vi "OLED.vi"() -> ()   [LabVIEW 2017]
uses:
  EnumEstados1.ctl
  <vilib>/Analysis/3filter.llb/Filter Passband Type.ctl
  <vilib>/Analysis/baseanly.llb/IIR Cascade Filter (DBL).vi
  <vilib>/Analysis/NI_AALBase.lvlib
panel:
  in  "Reiniciar":bool caption="Blank Button"
  in  "order":i32
  in  "Stop Button":bool
  in  "Save Button":bool
  in  "Guardar en:":path
  out "Voltage-Current Characterization:":cluster{dbl[], "Filtered X":dbl[]}(graph)
  in  "Ok":bool
  out "Voltaje de corte":dbl
  in  "Voltaje final:":dbl=5.0
  in  "Voltaje inicial:":dbl
  in  "Paso":dbl=0.1
  # "OLED"
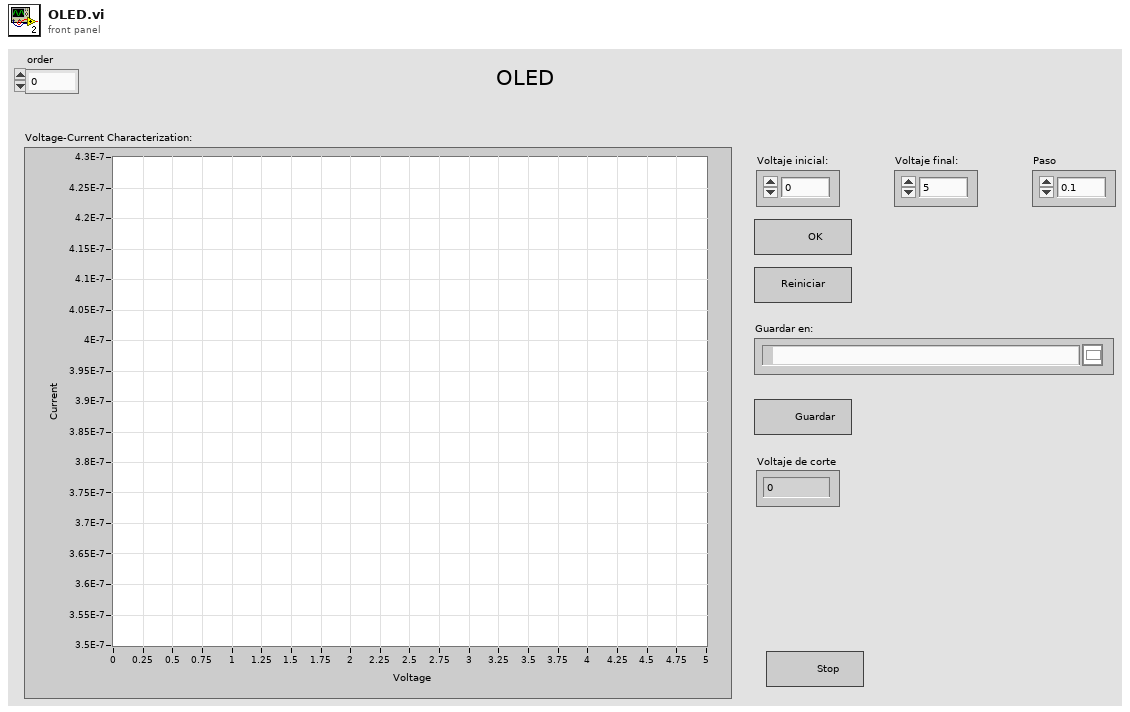
[diagram p1: front panel]
types:
  T1 = typedef "EnumEstados1.ctl" = enum16{"Inicio", "LecturaDatos", "Cierre"}
  T2 = typedef "NI_AALBase.lvlib/Filter Passband Type.ctl" = enum32{"Lowpass", "Highpass", "Bandpass", "Bandstop"}
  T3 = cluster{"task out":refnum<k21>, "error out":errorcluster}
  T4 = cluster{"filter structure":enum32{"IIR 2nd Order", "IIR 4th Order"}, "Reverse Coefficients":dbl[], "Forward Coefficients":dbl[]}
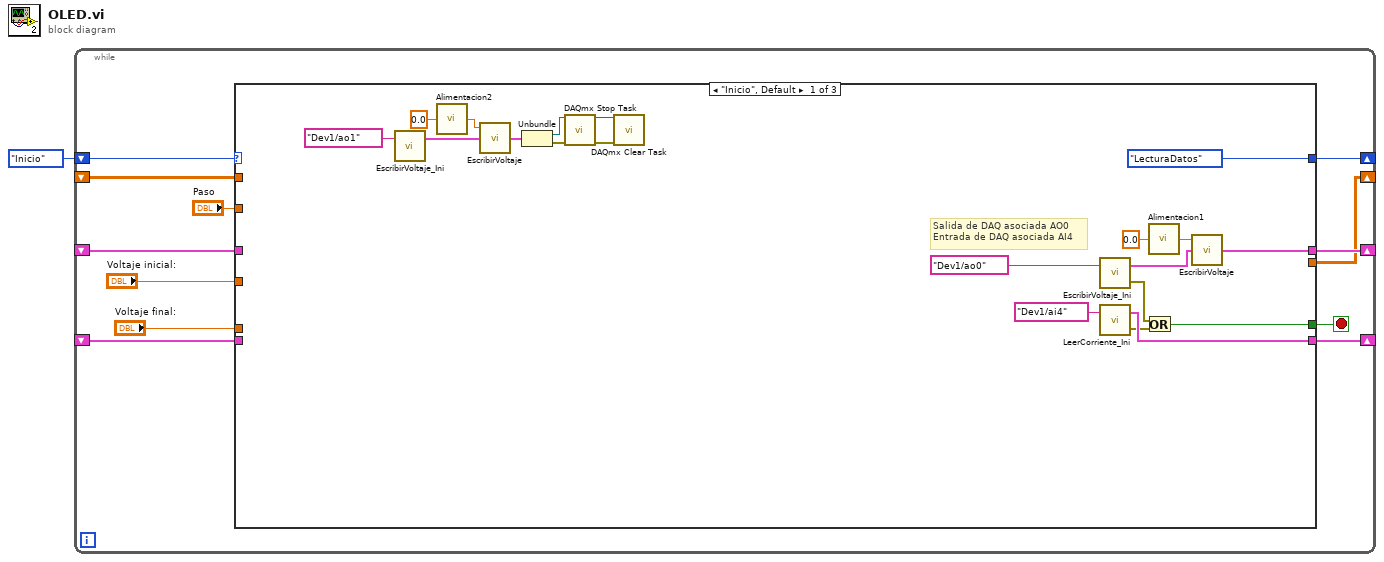
[diagram p0: block diagram]
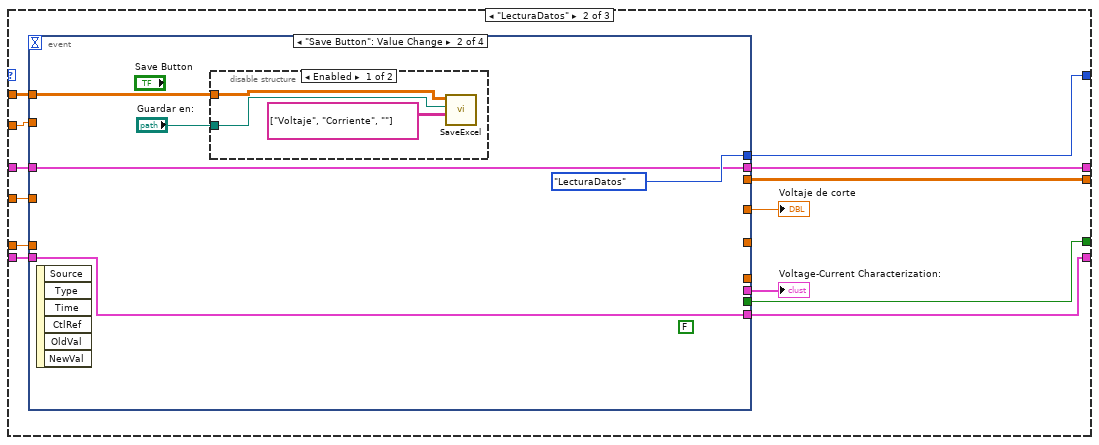
[diagram p2: hidden frame]
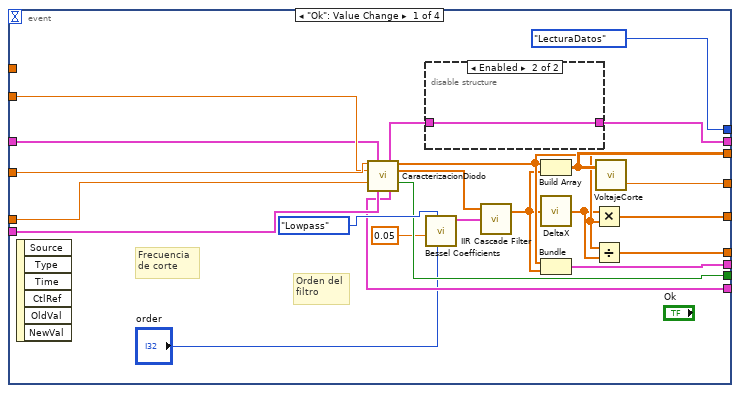
[diagram p3: hidden frame]
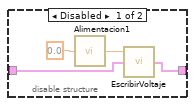
[diagram p4: hidden frame]
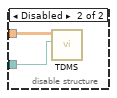
[diagram p5: hidden frame]
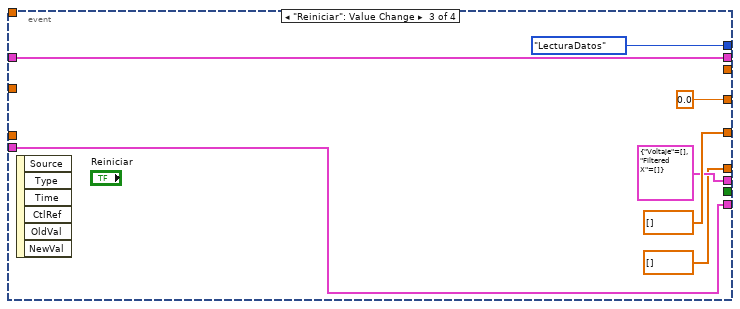
[diagram p6: hidden frame]
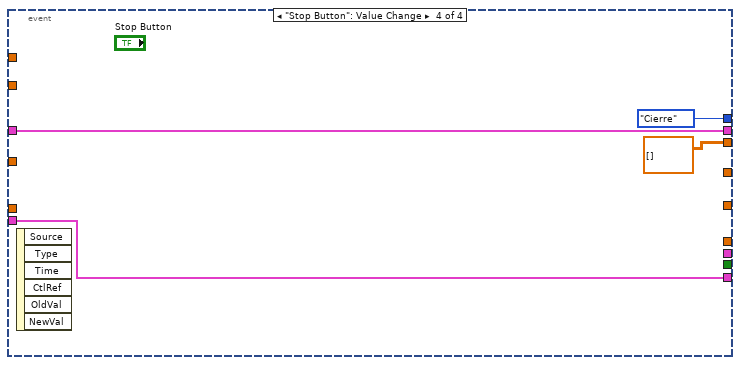
[diagram p7: hidden frame]
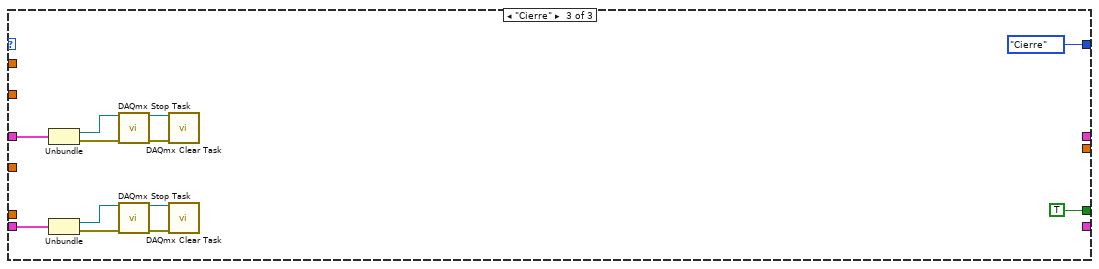
[diagram p8: hidden frame]
diagram:
  n1 = while {
    shift-right: [w5] -> _
    shift-left: EnumEstados1."Inicio" -> [w13]
    shift-right: [w9] -> _
    shift-left: _ -> [w8]
    shift-right: [w7] -> _
    shift-left: _ -> [w6]
    shift-right: [w4] -> _
    shift-left: _ -> [w3]
    stop <- w2 stop-if-true
    n2 = case shown="\"Inicio\", Default" w13 {
      tunnel: "Voltaje final:" -> [_ w46 _]
      tunnel: "Voltaje inicial:" -> [_ w40 _]
      tunnel: "Paso" -> [_ w41 _]
      tunnel: [w25 w44 _] -> w9
      tunnel: w8 -> [_ w45 w103]
      tunnel: [w32 w42 _] -> w7
      tunnel: w6 -> [_ w43 w102]
      tunnel: [EnumEstados1."LecturaDatos" w39 EnumEstados1."Cierre"] -> w5
      tunnel: [_ w38 _] -> w4
      tunnel: w3 -> [_ w37 _]
      tunnel: [w30 w36 TRUE] -> w2
      frame "Inicio", Default {
        # "Salida de DAQ asociada AO0\nEntrada de DAQ asociada AI4"
        n3 = call "EscribirVoltaje_Ini.vi"("physical channels"=tag "Dev1/ao1") -> ("cluster"=w21:T3)  [unwired: 1 in, 1 out]
        n4 = call "Alimentacion2.vi"("VoltajeDeseado"=0.0) -> ("Numeric Indicator"=w22:dbl)
        n5 = call "EscribirVoltaje.vi"("cluster"=w21, "data"=w22) -> ("Cluster"=w18:T3)  [unwired: 1 in, 2 out]
        n6 = Unbundle(w18) -> ("task out"=w17:refnum<k21>, "error out"=w16:errorcluster)
        n7 = call <vilib>:"DAQmx Stop Task.vi"("task/channels in"=w17, "error in"=w16) -> ("task out"=w20:refnum<k21>, "error out"=w19:errorcluster)  [unwired: 12 in]
        n8 = call <vilib>:"DAQmx Clear Task.vi"("task in"=w20, "error in"=w19) -> ()  [unwired: 13 in, 1 out]
        n9 = call "EscribirVoltaje_Ini.vi"("physical channels"=tag "Dev1/ao0") -> ("error out"=w24:errorcluster, "cluster"=w26:T3)  [unwired: 1 in]
        n10 = call "LeerCorriente_Ini.vi"("physical channels"=tag "Dev1/ai4") -> ("error out"=w31:errorcluster, "output cluster"=w32:T3)  [unwired: 1 in]
        n11 = Or(x=w24, y=w31) -> (x .or. y?=w30:bool)
        n12 = call "Alimentacion1.vi"("VoltajeDeseado"=0.0) -> ("Numeric Indicator"=w27:dbl)
        n13 = call "EscribirVoltaje.vi"("cluster"=w26, "data"=w27) -> ("Cluster"=w25:T3)  [unwired: 1 in, 2 out]
      }
      frame "LecturaDatos" {
        n14 = event shown="[1] \"Save Button\": Value Change" {
          selector: _ -> [_ _ _ _]
          dyn-events: _ -> [_ _ _ _]
          timeout: _ -> [_ _ _ _]
          tunnel: w46 -> [w63 _ _ _]
          tunnel: w45 -> [w62 w77 w86 w95]
          tunnel: [w67 w77 w86 w95] -> w44
          tunnel: w43 -> [w61 w76 w85 w94]
          tunnel: [w59 w76 w85 w94] -> w42
          tunnel: w41 -> [w64 _ _ _]
          tunnel: w40 -> [w65 _ _ _]
          tunnel: [EnumEstados1."LecturaDatos" EnumEstados1."LecturaDatos" EnumEstados1."LecturaDatos" EnumEstados1."Cierre"] -> w39
          tunnel: [w57 _ _ dbl[][] []] -> w38
          tunnel: w37 -> [_ w75 _ _]
          tunnel: [w58 _ _ _] -> w36
          tunnel: [w50 _ 0.0 ("Voltaje de corte") _] -> w35
          tunnel: [w49 _ dbl[] [] _] -> _
          tunnel: [w48 _ dbl[] [] _] -> _
          tunnel: [w47 _ cluster{"Voltaje":dbl[], "Filtered X":dbl[]} {"Voltaje"=[], "Filtered X"=[]} _] -> w34
          event "Ok": Value Change {
            # "Frecuencia \nde corte"
            # "Orden del\nfiltro"
            n15 = event-data() -> ()  [unwired: 1 in, 6 out]
            n16 = call "CaracterizacionDiodo.vi"("Voltaje inicial:"=w65, "Voltaje"=w62, "Paso"=w64, "Voltaje final:"=w63, "Corriente"=w61) -> (3:"Voltaje"=w60:T3, 4:"Voltaje"=w55:dbl[], 6:"Corriente"=w56:dbl[], "Error?"=w58:bool, 14:"Corriente"=w59:T3)  [unwired: 6 in]
            n17 = disable-structure shown="Enabled" {
              disable-tunnel: [w73 w74] -> w67
              disable-tunnel: w60 -> [w72 w74]
              frame Disabled {
                n18 = call "Alimentacion1.vi"("VoltajeDeseado"=0.0) -> ("Numeric Indicator"=w70:dbl)
                n19 = call "EscribirVoltaje.vi"("cluster"=w72, "data"=w70) -> ("Cluster"=w73:T3)  [unwired: 1 in, 2 out]
              }
              frame Enabled {
              }
            }
            n20 = call <vilib>:"Bessel Coefficients.vi"("order"="order", "filter type"=Filter_Passband_Type."Lowpass", "low cutoff freq: fl"=0.05 ("Numeric Control")) -> ("IIR Filter Cluster"=w69:T4)  [unwired: 7 in, 1 out]
            n21 = call-poly <vilib>:"IIR Cascade Filter.vi"("IIR Filter Cluster"=w69, "X"=w56) -> ("Filtered X"=w53:dbl[])  [unwired: 1 in, 1 out]
            n22 = Build Array(w55, w53) -> (w57:dbl[][])
            n23 = call "DeltaX.vi"("Array in"=w53) -> ("Array out"=w54:dbl[])
            n24 = Bundle("Voltaje"=w55, "Filtered X"=w53) -> (w47:cluster{"Voltaje":dbl[], "Filtered X":dbl[]})  [unwired: 1 in]
            n25 = Multiply(x=w54, y=w55) -> (x*y=w49:dbl[])
            n26 = Divide(x=w55, y=w54) -> (x/y=w48:dbl[])
            n27 = call "VoltajeCorte.vi"("Array in"=w57) -> ("Voltaje de corte"=w50:dbl)  [unwired: 1 in, 1 out]
          }
          event "Save Button": Value Change {
            (unwired) FALSE
            n28 = event-data() -> ()  [unwired: 1 in, 6 out]
            n29 = disable-structure shown="Enabled" {
              disable-tunnel: "Guardar en:" -> [w81 w84]
              disable-tunnel: w75 -> [w82 w83]
              frame Enabled {
                n30 = call "SaveExcel.vi"("Array 2"=string[][] [["Voltaje", "Corriente", ""]], "Guardar en:"=w81, "Array"=w82) -> ()  [unwired: 9 in]
              }
              frame Disabled {
                n31 = call "TDMS.vi"("Guardar en:"=w84, "Array"=w83) -> ()  [unwired: 10 in]
              }
            }
          }
          event "Reiniciar": Value Change {
            n32 = event-data() -> ()  [unwired: 1 in, 6 out]
          }
          event "Stop Button": Value Change {
            n33 = event-data() -> ()  [unwired: 1 in, 6 out]
          }
        }
        "Voltaje de corte" <- w35
        "Voltage-Current Characterization:" <- w34
      }
      frame "Cierre" {
        n34 = Unbundle(w103) -> ("task out"=w101:refnum<k21>, "error out"=w100:errorcluster)
        n35 = Unbundle(w102) -> ("task out"=w99:refnum<k21>, "error out"=w98:errorcluster)
        n36 = call <vilib>:"DAQmx Stop Task.vi"("task/channels in"=w101, "error in"=w100) -> ("task out"=w107:refnum<k21>, "error out"=w106:errorcluster)  [unwired: 12 in]
        n37 = call <vilib>:"DAQmx Stop Task.vi"("task/channels in"=w99, "error in"=w98) -> ("task out"=w105:refnum<k21>, "error out"=w104:errorcluster)  [unwired: 12 in]
        n38 = call <vilib>:"DAQmx Clear Task.vi"("task in"=w107, "error in"=w106) -> ()  [unwired: 13 in, 1 out]
        n39 = call <vilib>:"DAQmx Clear Task.vi"("task in"=w105, "error in"=w104) -> ()  [unwired: 13 in, 1 out]
      }
    }
  }
